vi "LVDimInterface.acquire.vi"(3 "ms timeout (10000)":i32=10000, 5 "error in (no error)":errorcluster) -> (17 "timed out":bool, 19 "error out":errorcluster)   [LabVIEW 2015, in "LVDimInterface.lvlib"]
doc: "Acquires (locks) the LVDimInterface for changes. This routine is intended for internal purposes only.\n\nLicense Agreement for this software:\n\nCopyright (C)\nGesellschaft für Schwerionenforschung, GSI\nPlanckstr. 1\n64291 Darmstadt\nGermany\n\nContact: D.Beck@gsi.de \n\nThis program is free software; you can redistribute it and/or modify it under the terms of the GNU General Public License as published by the Free Software Foundation; either version 2 of the license, or (at your option) any later version.\n\nThis program is distributed in the hope that it will be useful, but WITHOUT ANY WARRANTY; without even the implied warranty of MERCHANTABILITY or FITNESS FOR A PARTICULAR PURPOSE. See the GNU General License for more details (http://www.gnu.org).\n\nGesellschaft für Schwerionenforschung, GSI\nPlanckstr. 1, 64291 Darmstadt, Germany\nFor all questions and ideas contact: M.Richter@gsi.de, H.Brand@gsi.de or D.Beck@gsi.de.\nLast update: 17-JUN-2004"
uses:
  LVDimInterface.lvlib
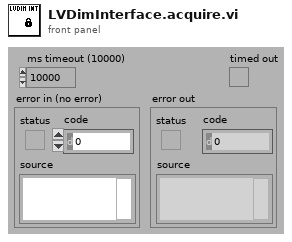
[diagram p1: front panel]
types:
  T1 = enum16{"unknown", "createSemaphore", "destroySemaphore", "getSemaphore"}
  T2 = typedef "Semaphore RefNum" = refnum<k1>
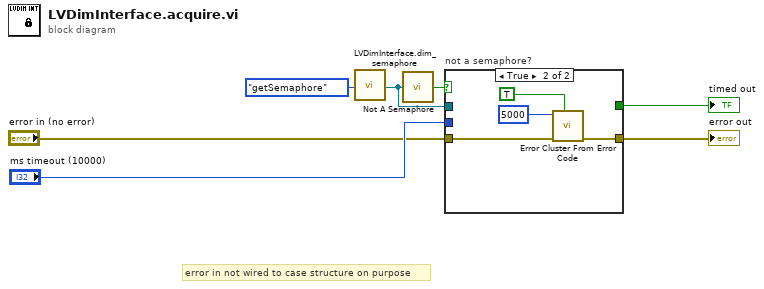
[diagram p0: block diagram]
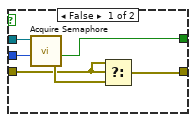
[diagram p2: hidden frame]
diagram:
  # "error in not wired to case structure on purpose"
  n1 = call "LVDimInterface.dim_semaphore.vi"("Action"=T1."getSemaphore") -> ("semaphore"=w1:T2)  [unwired: 18 in]
  n2 = call <vilib>:"Not A Semaphore.vi"("semaphore"=w1) -> ("not a semaphore"=w3:bool)
  n3 = case "not a semaphore?" shown="True" w3 {
    tunnel: [w13 _] -> w7
    tunnel: "ms timeout (10000)" -> [w12 _]
    tunnel: [w11 w16] -> w5
    tunnel: w1 -> [w10 _]
    tunnel: "error in (no error)" -> [w8 w17]
    frame False {
      n4 = call <vilib>:"Acquire Semaphore.vi"("ms timeout (-1)"=w12, "semaphore"=w10) -> ("error out"=w9:errorcluster, "timed out"=w13:bool)  [unwired: 3 in, 1 out]
      n5 = Select(t=w8, s=w8, f=w9) -> (s? t:f=w11:errorcluster)
    }
    frame True {
      n6 = call <vilib>:"Error Cluster From Error Code.vi"("show call chain? (False)"=TRUE, "error in (no error)"=w17, "error code (0)"=5000 ("code")) -> ("error out"=w16:errorcluster)  [unwired: 6 in]
    }
  }
  "error out" <- w5
  "timed out" <- w7
